vi "MH_OpenPTU.vi"(8 "entrée d'erreur":errorcluster) -> (0 "sortie d'erreur":errorcluster, 2 "Cancelled":bool, 3 "refnum en sortie":refnum<file>)   [LabVIEW 2019]
panel:
  out "Version":string
  out "Magic":string
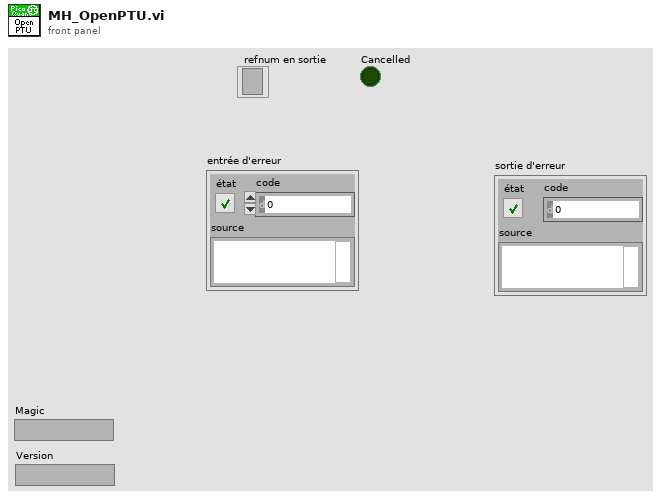
[diagram p1: front panel]
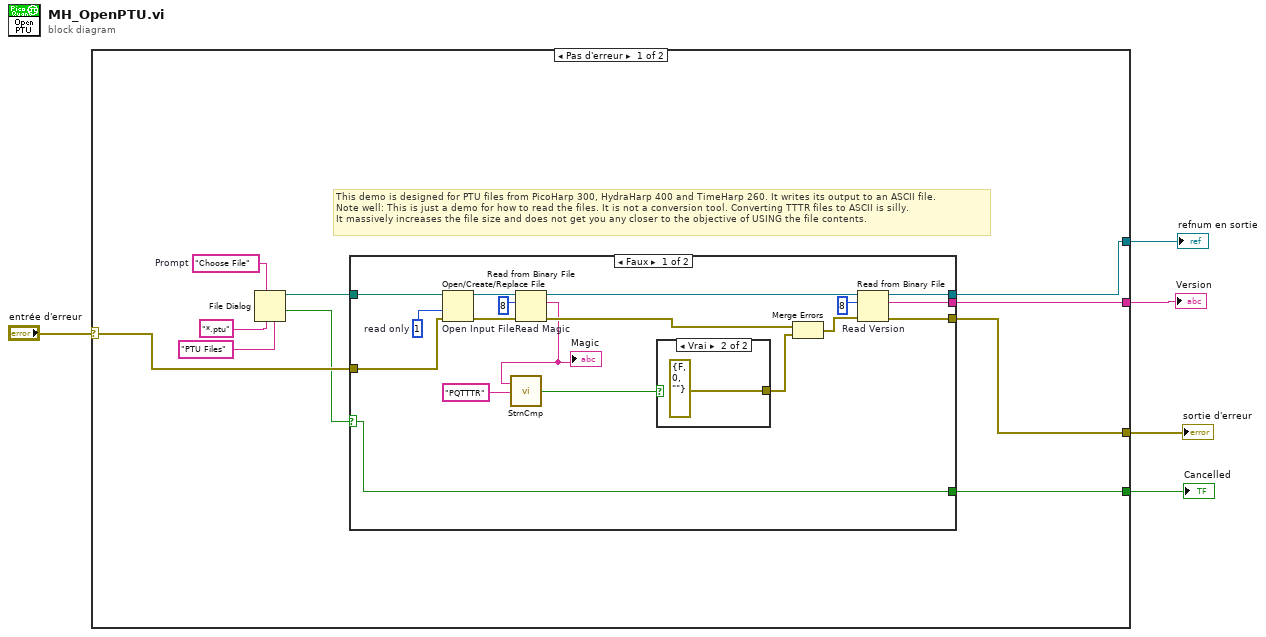
[diagram p0: block diagram]
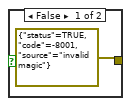
[diagram p2: hidden frame]
diagram:
  n1 = case shown="Pas d'erreur" "entrée d'erreur" {
    selector: "entrée d'erreur" -> [w9 w38]
    tunnel: [w11 _] -> w5
    tunnel: [w10 w38] -> w4
    tunnel: [w8 _] -> w2
    tunnel: [w6 _] -> w1
    frame No Error {
      w15 = "Choose File"  # Prompt
      # "This demo is designed for PTU files from PicoHarp 300, HydraHarp 400 and TimeHarp 260. It writes its output to an ASCII file.\nNote well: This is just a demo for how to read the files. It is not a conversion tool. Converting TTTR files to ASCII is silly.\nIt massively increases the file size and does not get you any closer to the objective of USING the file contents."
      n2 = File Dialog(4:"PTU Files", 6:"*.ptu", 7:w15) -> (1:w7:bool, 3:w12:path)  [unwired: 4 in, 2 out]
      n3 = case shown="Faux" w7 {
        selector: w7 -> [w16 w36]
        tunnel: w12 -> [w22 _]
        tunnel: [w20 _] -> w11
        tunnel: [w19 w37] -> w10
        tunnel: w9 -> [w18 w37]
        tunnel: [w17 _] -> w8
        tunnel: [w16 w36] -> w6
        frame False {
          w21 = 1  # read only
          n4 = Open/Create/Replace File "Open Input File"(file path (use dialog)=w22, error in=w18, access (0:read/write)=w21) -> (refnum out=w25:refnum<file>, error out=w24:errorcluster)  [unwired: 3 in, 1 out]
          n5 = Read from Binary File "Read Magic"(8:w24, 10:8, 11:w25) -> (0:w30:errorcluster, 2:w26:string, 3:w33:refnum<file>)  [unwired: 3 in, 1 out]
          "Magic" <- w26
          n6 = call "StrnCmp.vi"("String 2"="PQTTTR", "String 1"=w26) -> ("equal"=w27:bool)
          n7 = case shown="Vrai" w27 {
            tunnel: [errorcluster {"status"=TRUE, "code"=-8001, "source"="invalid magic"} ("file error status 2") errorcluster {"status"=FALSE, "code"=0, "source"=""} ("file error status 2")] -> w28
            frame False {
            }
            frame True {
            }
          }
          n8 = Merge Errors(w30, w28) -> (w29:errorcluster)
          n9 = Read from Binary File "Read Version"(8:w29, 10:8, 11:w33) -> (0:w19:errorcluster, 2:w20:string, 3:w17:refnum<file>)  [unwired: 3 in, 1 out]
        }
        frame True {
        }
      }
    }
    frame Error {
    }
  }
  "Version" <- w5
  "sortie d'erreur" <- w4
  "refnum en sortie" <- w2
  "Cancelled" <- w1
